vi "set_bounding_box.vi"(8 "error in (no error)":errorcluster, 9 "new size":refnum<class "SpaceVector.lvclass">, 10 "new center":refnum<class "SpaceVector.lvclass">, 11 "RoiGeneric in":refnum<class "RoiGeneric.lvclass">) -> (0 "error out":errorcluster, 3 "RoiGeneric out":refnum<class "RoiGeneric.lvclass">)   [LabVIEW 2010, in "RoiGeneric.lvclass"]
uses:
  RoiGeneric.lvclass
  common/classes/SpaceVector/SpaceVector/SpaceVector.lvclass
  RoiGeneric.lvclass/RoiGeneric.ctl
  common/classes/Box/Box/Box.lvclass
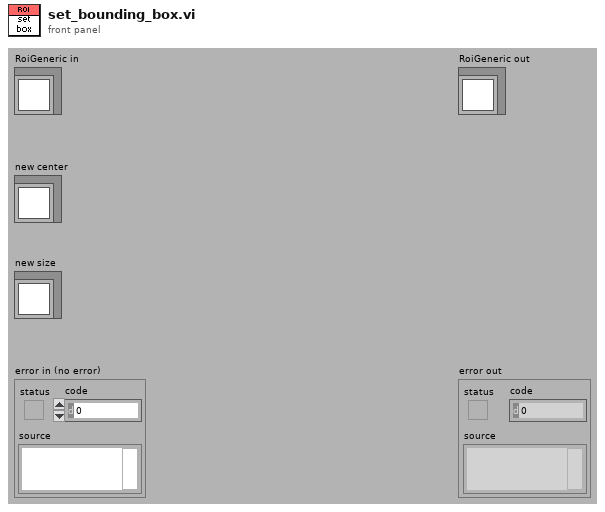
[diagram p1: front panel]
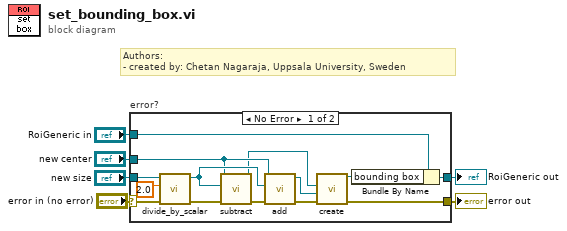
[diagram p0: block diagram]
diagram:
  # "Authors: \n- created by: Chetan Nagaraja, Uppsala University, Sweden"
  n1 = case "error?" shown="No Error" "error in (no error)" {
    selector: "error in (no error)" -> [w10 w22]
    tunnel: [w18 w22] -> w5
    tunnel: [w19 w21] -> w3
    tunnel: "RoiGeneric in" -> [w20 w21]
    tunnel: "new size" -> [w9 _]
    tunnel: "new center" -> [w11 _]
    frame No Error {
      n2 = call "divide_by_scalar.vi"("error in (no error)"=w10, "divisor"=2.0, "SpaceVector in"=w9) -> ("error out"=w15:errorcluster, "SpaceVector out"=w13:refnum<class "SpaceVector.lvclass">)  [unwired: 7 in]
      n3 = call "subtract.vi"("error in (no error)"=w15, "subtrahend"=w13, "SpaceVector in"=w11) -> ("error out"=w14:errorcluster, "SpaceVector out"=w7:refnum<class "SpaceVector.lvclass">)  [unwired: 7 in]
      n4 = call "add.vi"("error in (no error)"=w14, "vector to be added"=w13, "SpaceVector in"=w11) -> ("error out"=w12:errorcluster, "SpaceVector out"=w8:refnum<class "SpaceVector.lvclass">)  [unwired: 7 in]
      n5 = call "create.vi"("error in (no error)"=w12, "maximum"=w8, "minimum"=w7) -> ("error out"=w18:errorcluster, "Box out"=w17:refnum<class "Box.lvclass">)  [unwired: 7 in]
      n6 = Bundle By Name(cluster=w20, "bounding box"=w17) -> (w19:refnum<class "RoiGeneric.lvclass">)
    }
    frame Error {
    }
  }
  "error out" <- w5
  "RoiGeneric out" <- w3
